vi "Get Local Destination Path.vi"(8 "error in (no error)":errorcluster, 11 "NI_AB_API_DPPL in":refnum<class "NI_AB_API_DPPL.lvclass">) -> (0 "error out":errorcluster, 2 "Local destination path":path, 3 "NI_AB_API_DPPL out":refnum<class "NI_AB_API_DPPL.lvclass">)   [LabVIEW 2020, in "NI_AB_API_DPPL.lvclass"]
uses:
  <vilib>/AppBuilder/AB_API/DPPL/NI_AB_API_DPPL.lvclass
  <vilib>/AppBuilder/AB_API/DPPL/NI_AB_API_DPPL.lvclass/NI_AB_API_DPPL.ctl
  <vilib>/AppBuilder/AB_API/Build/NI_AB_API_Build.lvclass
  <vilib>/AppBuilder/AB_Classes/Build/AB_Build.lvclass
  e:/builds/penguin/labview/branches/2020/dev/dist/vi.lib/AppBuilder/AB_API/PPL/NI_AB_API_PPL.lvclass
  e:/builds/penguin/labview/branches/2020/dev/dist/vi.lib/AppBuilder/AB_API/Targetfile/NI_AB_API_Targetfile.lvclass
  e:/builds/penguin/labview/branches/2020/dev/dist/vi.lib/AppBuilder/AB_API/Build/NI_AB_API_Build.lvclass
  e:/builds/penguin/labview/branches/2020/dev/dist/vi.lib/AppBuilder/AB_API/DPPL/NI_AB_API_DPPL.lvclass
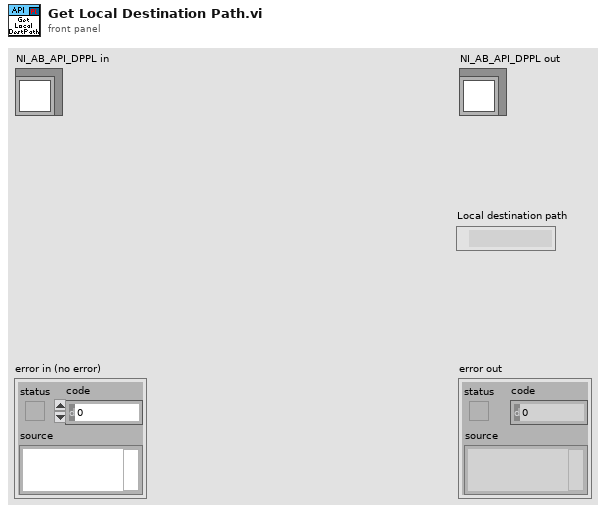
[diagram p1: front panel]
types:
  T1 = typedef "AB_Build.ctl" = cluster{"buildSpecName":string, "buildSpecDescription":string, "destinations":refnum<class "AB_Destination.lvclass">[], "exclusionOption":T2, "defaultLanguage":string, "supportedLanguages":string[], "excludedDirectories":path[], "buildContext":refnum<vi>, "buildObject":T3, "preview":bool, "programatic":bool, "progressBarEvents":T4, "userLog_Path":path, "preActionID":string, "preAction_Path":path, "postActionID":string, "postAction_Path":path, "eng_checkForBrokenVIs?":bool, "eng_verboseLinkerErrors?":bool, "localDest_Path":path, "targetDest_Path":path, "removeVIObject":u16, "cache":refnum<class "PreviewCache.lvclass">, "use cache":bool, "previewCache_ID":string, "buildCache_ID":string, "eng_TempLocalDest_Path":path, "eng_collectDependencies?":bool, "versionInfo":cluster{"buildVersion":cluster{"major":u16, "minor":u16, "patch":u16, "build":u16}, "autoIncrement":bool}, "eng_enableVIChecksums":bool}
  T2 = typedef "AB_Exclusion_Option.ctl" = cluster{"typedefs":bool, "polymorphicVIs":bool, "unusedLibraryItems":bool, "modifyLibraryFile":bool, "edit-timeDependencies":bool, "inlineVIs":bool, "dependent PPLs":bool, "dependent DLLs":bool}
  T3 = typedef "ItemRef.ctl" = u64
  T4 = typedef "provcom_ProgressBar_Events.ctl" = cluster{"newJob":refnum<user-event>, "newItem":refnum<user-event>, "errorMsg":T5, "cancel":refnum<user-event>}
  T5 = typedef "mxLvBuildError.ctl" = refnum<user-event>
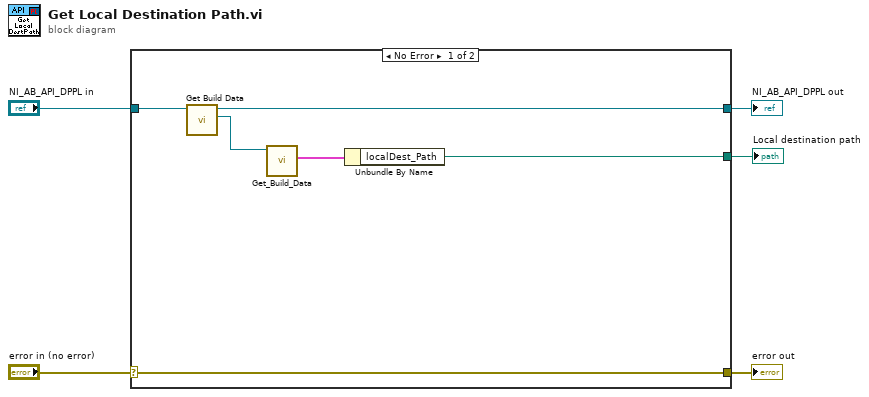
[diagram p0: block diagram]
diagram:
  n1 = case shown="No Error" "error in (no error)" {
    selector: "error in (no error)" -> [w11 w13]
    tunnel: [w11 w13] -> w4
    tunnel: [w7 w12] -> w2
    tunnel: "NI_AB_API_DPPL in" -> [w8 w12]
    tunnel: [w6 _] -> w1
    frame No Error {
      n2 = call <vilib>:"Get Build Data.vi"("NI_AB_API_Build in"=w8) -> ("AB_Build.lvclass"=w10:refnum<class "AB_Build.lvclass">, "NI_AB_API_Build out"=w7:refnum<class "NI_AB_API_DPPL.lvclass">)  [unwired: 8 in, 1 out]
      n3 = call <vilib>:"Get_Build_Data.vi"("Class in"=w10) -> ("data"=w9:T1)  [unwired: 8 in, 2 out]
      n4 = Unbundle By Name(w9) -> ("localDest_Path"=w6:path)
    }
    frame Error {
    }
  }
  "error out" <- w4
  "NI_AB_API_DPPL out" <- w2
  "Local destination path" <- w1
